vi "Get Modifier.vi"(0 "Modifier Code":i16) -> (1 "Modifiers":T1[](array[typedef]), 2 "Modifiers Concatenated":string)   [LabVIEW 2021, in "Seq Edit Quick Drop.lvlib"]
uses:
  Seq Edit Quick Drop.lvlib
  Modifiers.ctl
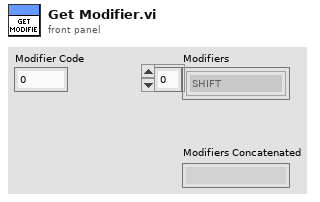
[diagram p1: front panel]
types:
  T1 = typedef "Seq Edit Quick Drop.lvlib/Modifiers.ctl" = enum16{"SHIFT", "CTRL", "ALT"}
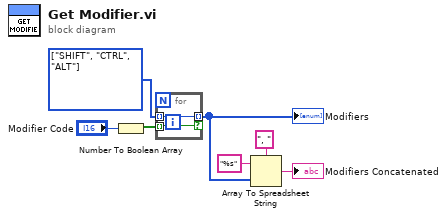
[diagram p0: block diagram]
diagram:
  w6 = T1[] [enum."SHIFT", enum."CTRL", enum."ALT"] items=["SHIFT", "CTRL", "ALT"]
  n1 = Number To Boolean Array(number="Modifier Code") -> (Boolean array=w5:bool[])
  n2 = for {
    tunnel: w5 -> [w8] mode=indexing
    tunnel: w6 -> [w9] mode=indexing
    tunnel: [w9] -> w4 mode=indexing if=w8
  }
  "Modifiers" <- w4
  n3 = Array To Spreadsheet String(delimiter (Tab)=", ", array=w4, 3:"%s" ("format string")) -> (spreadsheet string=→"Modifiers Concatenated":string)
